vi "Display.vi"(8 "error in (no error)":errorcluster, 11 "MQTT-Server in":refnum<class "MQTT-Server.lvclass">) -> (0 "error out":errorcluster, 2 "Waveform[]":waveform(dbl)[](array[waveform]), 3 "MQTT-Server out":refnum<class "MQTT-Server.lvclass">)   [LabVIEW 2023, in "MQTT-Server.lvlib" / "MQTT-Server.lvclass"]
uses:
  MQTT-Server.lvclass
  MQTT-Server.lvclass/MQTT-Server.ctl
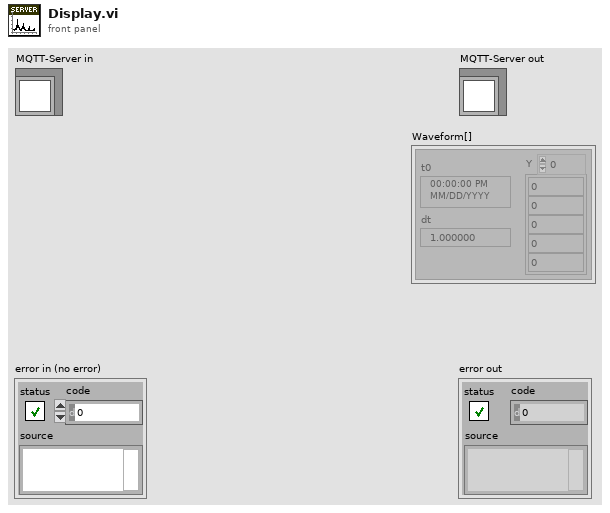
[diagram p1: front panel]
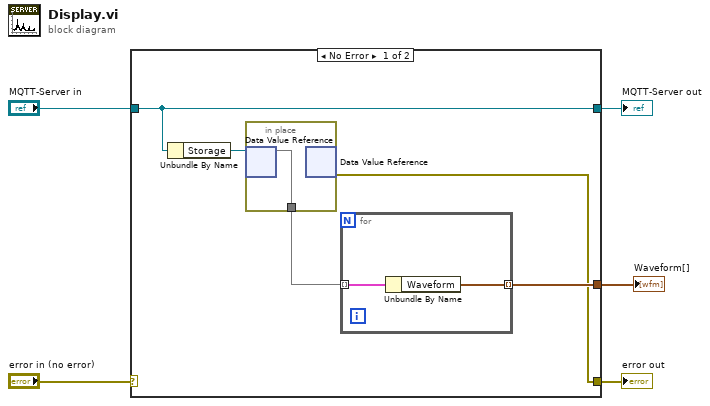
[diagram p0: block diagram]
diagram:
  n1 = case shown="No Error" "error in (no error)" {
    selector: "error in (no error)" -> [_ w15]
    tunnel: [w6 w15] -> w4
    tunnel: [w10 w14] -> w2
    tunnel: "MQTT-Server in" -> [w10 w14]
    tunnel: [w7 _] -> w1
    frame No Error {
      n2 = Unbundle By Name(w10) -> ("Storage"=w9:refnum<data-value>)
      n3 = in-place {
        in-place-border: [w13] -> w8
        n4 = in-place-dvr #1(w9) -> (w13:map{string, waveform(dbl)})  [unwired: 1 out]
        n5 = in-place-dvr #1() -> (w6:errorcluster)  [unwired: 1 in, 1 out]
      }
      n6 = for {
        tunnel: w8 -> [w12] mode=indexing
        tunnel: [w11] -> w7 mode=indexing
        n7 = Unbundle By Name(w12) -> ("Waveform"=w11:waveform(dbl))
      }
    }
    frame Error {
    }
  }
  "error out" <- w4
  "MQTT-Server out" <- w2
  "Waveform[]" <- w1
